vi "Send Add Data with TS.vi"(0 "Message Enqueuer":refnum<class "Message Enqueuer.lvclass">, 1 "Time Stamp":timestamp format="%<%x %.3X>T", 2 "Values":dbl[](array[numeric]), 5 "error in (no error)":errorcluster, 6 "Actor Name":string, 7 "Callback Queue":refnum<queue>, 8 "Message Priority (Normal)":T1=enum."Normal", 9 "timeout in ms (-1)":i32) -> (13 "TimeOut":bool, 14 "Message Enqueuer out":refnum<class "Message Enqueuer.lvclass">, 19 "error out":errorcluster)   [LabVIEW 2018, in "BNT_XtGraph.lvlib" / "Add Data with TS Msg.lvclass"]
doc: "Sends the <B>BNT_XtGraph.lvlib:Add Data with TS Msg.lvclass</B> message.\n\n<B>BNT_XtGraph.lvlib:BNT_XtGraph.lvclass:Add Data with TS.vi</B> Description:\n\nAdd actual data with one timestamp for all channels to history."
uses:
  Add Data with TS Msg.lvclass
  <vilib>/ActorFramework/Message Enqueuer/Message Enqueuer.lvclass
  <vilib>/ActorFramework/Message Enqueuer/Message Priority.ctl
  C:/Users/Holger/Documents/LVP/HEITRONICS/TempCtrl/Packages/CSPP_Core/Messages/CSPP_AsyncCallbackMsg/CSPP_AsyncCallback Msg.lvclass
  C:/Program Files (x86)/National Instruments/LabVIEW 2018/vi.lib/ActorFramework/Message/Message.lvclass
  Add Data with TS Msg.lvclass/Add Data with TS Msg.ctl
  CSPP_Core/Messages/CSPP_AsyncCallbackMsg/CSPP_AsyncCallback Msg.lvclass/CSPP_AsyncCallback Msg.ctl
  <vilib>/ActorFramework/Message Enqueuer/Message Enqueuer.lvclass/Message Enqueuer.ctl
  <vilib>/ActorFramework/Message Priority Queue/Priority Enqueue.vi
  CSPP_Core/Messages/CSPP_AsyncCallbackMsg/CSPP_AsyncCallback Msg.lvclass
  CSPP_Core/Libraries/Utilities/CSPP_Utilities.lvlib
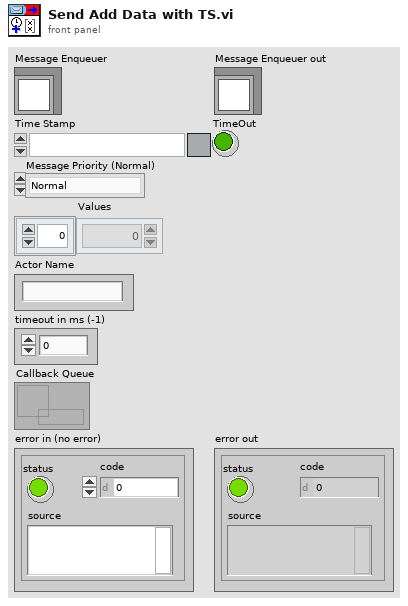
[diagram p1: front panel]
types:
  T1 = typedef "Actor Framework.lvlib/Message Enqueuer.lvclass/Message Priority.ctl" = enum16{"Low", "Normal", "High"}
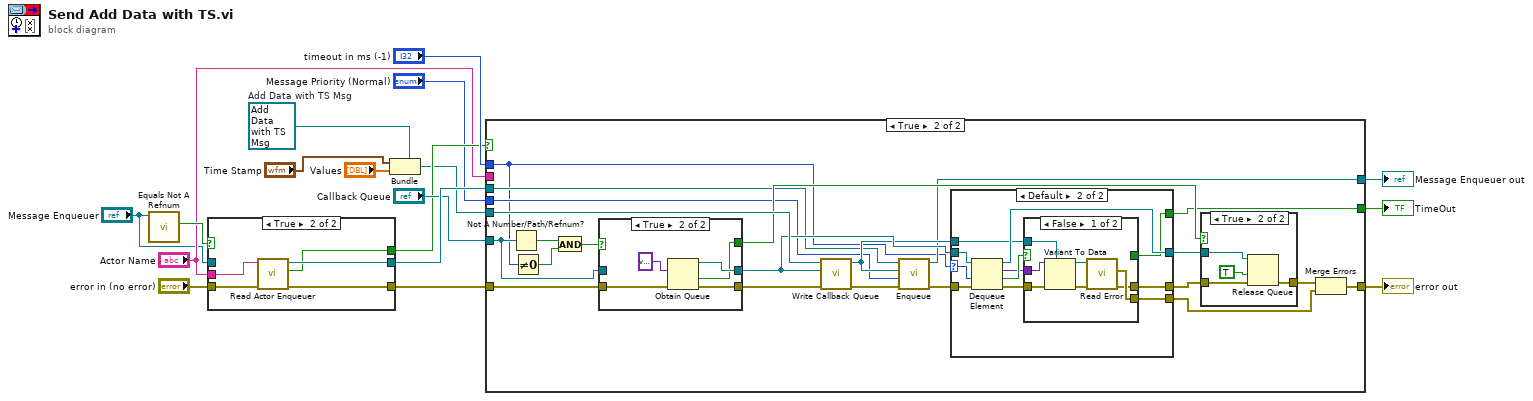
[diagram p0: block diagram]
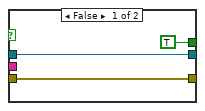
[diagram p2: hidden frame]
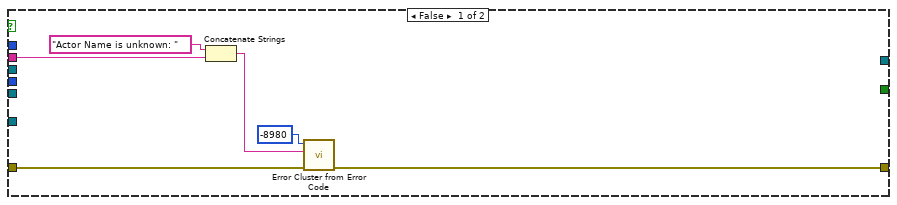
[diagram p3: hidden frame]
diagram:
  w4 = refnum<class "Add Data with TS Msg.lvclass"> refnum  # Add Data with TS Msg
  n1 = call <vilib>:"Equals Not A Refnum.vi"("Message Enqueuer"="Message Enqueuer") -> ("Not a refnum?"=w17:bool)  [unwired: 10 in]
  n2 = case shown="True" w17 {
    tunnel: "error in (no error)" -> [w19 w25]
    tunnel: [w19 w24] -> w16
    tunnel: "Actor Name" -> [_ w21]
    tunnel: [w20 w23] -> w15
    tunnel: "Message Enqueuer" -> [w20 _]
    tunnel: [TRUE ("Success") w22] -> w11
    frame False {
    }
    frame True {
      n3 = call "Read Actor Enqueuer.vi"("Error In"=w25, "Actor Name"=w21) -> ("Error Out"=w24:errorcluster, "Success"=w22:bool, "Enqueuer"=w23:refnum<class "Message Enqueuer.lvclass">)  [unwired: 6 in, 1 out]
    }
  }
  n4 = Bundle ("Main-Bundle")(cluster=w4, "Time Stamp", "Values") -> (w5:refnum<class "Add Data with TS Msg.lvclass">)
  n5 = case shown="True" w11 {
    tunnel: w5 -> [_ w53]
    tunnel: w16 -> [w31 w42]
    tunnel: w15 -> [_ w41]
    tunnel: "Message Priority (Normal)" -> [_ w40]
    tunnel: "Callback Queue" -> [_ w33]
    tunnel: [_ w39] -> w7
    tunnel: [w30 w38] -> w8
    tunnel: [_ w37] -> w13
    tunnel: "timeout in ms (-1)" -> [_ w32]
    tunnel: "Actor Name" -> [w26 _]
    frame False {
      n6 = Concatenate Strings("Actor Name is unknown: " ("Error Message (\"\")"), w26) -> (w27:string)
      n7 = call "Error Cluster from Error Code.vi"("Error In"=w31, "Error Message (\"\")"=w27, "Error Code (0)"=-8980) -> ("Error Out"=w30:errorcluster)  [unwired: 8 in]
    }
    frame True {
      n8 = Not A Number/Path/Refnum?(number/path/refnum=w33) -> (NaN/Path/Refnum?=w36:bool)
      n9 = Not Equal To 0?(x=w32) -> (x != 0?=w35:bool)
      n10 = And(x=w36, y=w35) -> (x .and. y?=w34:bool)
      n11 = case shown="True" w34 {
        tunnel: w33 -> [w77 _]
        tunnel: [w77 w82] -> w50
        tunnel: [w76 w80] -> w51
        tunnel: w42 -> [w76 w79]
        tunnel: [_ w78] -> w48
        frame False {
        }
        frame True {
          n12 = Obtain Queue(element data type=variant, error in (no error)=w79) -> (queue out=w82:refnum<queue>, created new?=w78:bool, error out=w80:errorcluster)  [unwired: 3 in]
        }
      }
      n13 = call "Write Callback Queue.vi"("error in (no error)"=w51, "Callback Queue"=w50, "CSPP_AsyncCallback Msg in"=w53) -> ("error out"=w52:errorcluster, "CSPP_AsyncCallback Msg out"=w44:refnum<class "Add Data with TS Msg.lvclass">)  [unwired: 7 in]
      n14 = call <vilib>:"Enqueue.vi"("error in (no error)"=w52, "Message Priority (Normal)"=w40, "Message"=w44, "Message Enqueuer in"=w41) -> ("error out"=w49:errorcluster, "Message Enqueuer out"=w39:refnum<class "Message Enqueuer.lvclass">)  [unwired: 6 in]
      n15 = case shown="Default" w32 {
        selector: w32 -> [_ w63]
        tunnel: w50 -> [w55 w64]
        tunnel: [w55 w66] -> w47
        tunnel: [w54 w56] -> w46
        tunnel: w49 -> [w54 w65]
        tunnel: w44 -> [_ w60]
        tunnel: [_ w58] -> w37
        tunnel: [_ w57] -> w43
        frame 0 {
        }
        frame Default {
          n16 = Dequeue Element(queue=w64, timeout in ms (-1)=w63, error in (no error)=w65) -> (queue out=w66:refnum<queue>, element=w61:variant, timed out?=w62:bool, error out=w59:errorcluster)
          n17 = case "Dequeue Case" shown="False" w62 {
            selector: w62 -> [_ w75]
            tunnel: w61 -> [w73 _]
            tunnel: w60 -> [w72 _]
            tunnel: w59 -> [w71 w74]
            tunnel: [_ w75] -> w58
            tunnel: [w68 _] -> w57
            tunnel: [w67 w74] -> w56
            frame False {
              n18 = Variant To Data(error in=w71, type=w72, Variant=w73) -> (data=w70:refnum<class "Add Data with TS Msg.lvclass">, error out=w69:errorcluster)
              n19 = call "Read Error.vi"("error in (no error)"=w69, "CSPP_AsyncCallback Msg in"=w70) -> ("error out"=w67:errorcluster, "Error"=w68:errorcluster)  [unwired: 7 in, 1 out]
            }
            frame True {
            }
          }
        }
      }
      n20 = case shown="True" w48 {
        tunnel: w47 -> [_ w87]
        tunnel: w46 -> [w83 w86]
        tunnel: [w83 w84] -> w45
        frame False {
        }
        frame True {
          n21 = Release Queue(queue=w87, force destroy? (F)=TRUE, error in (no error)=w86) -> (error out=w84:errorcluster)  [unwired: 2 out]
        }
      }
      n22 = Merge Errors(w45, w43) -> (w38:errorcluster)
    }
  }
  "error out" <- w8
  "Message Enqueuer out" <- w7
  "TimeOut" <- w13
